vi "lv_mysql_conn_encrypt_passwd.vi"(1 "Data":u8[](array[numeric]) format="%.0x", 2 "Scramble":u8[](array[numeric]) format="%.0x") -> (0 "SHA1 Data":u8[](array[numeric]) format="%.0x")   [LabVIEW 2010]
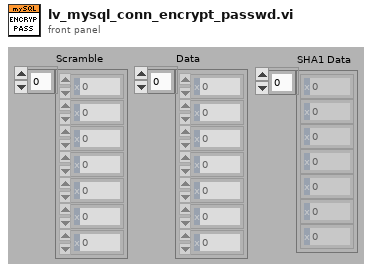
[diagram p1: front panel]
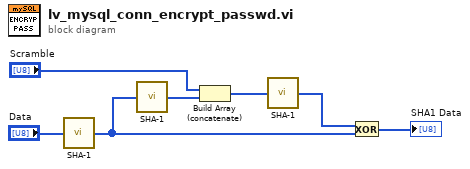
[diagram p0: block diagram]
diagram:
  n1 = call "SHA-1.vi"("Data"="Data") -> ("message-digest"=w6:u8[])
  n2 = call "SHA-1.vi"("Data"=w6) -> ("message-digest"=w4:u8[])
  n3 = Build Array (concatenate)("Scramble", w4) -> (w1:u8[])
  n4 = call "SHA-1.vi"("Data"=w1) -> ("message-digest"=w5:u8[])
  n5 = Exclusive Or(1:w6, 2:w5) -> (0:→"SHA1 Data":u8[])
